vi "TCP.vi"(11 "PortSettings":cluster{"IP Address":string, "Port":u16}) -> ()   [LabVIEW 2019]
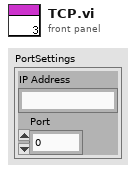
[diagram p1: front panel]
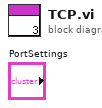
[diagram p0: block diagram]
diagram:
